vi "TimeTag_Nov 15_2022 - delay adjust.vi"() -> ()   [LabVIEW 2015]
doc: "This sample project is built upon the standard state machine template and shows how you could create an application that acquires, analyzes, and presents data. It includes functionality for presenting configuration dialogs, preserving settings between executions, loading and saving data, as well as exporting graph images and text files.\n\nIt is most appropriate for data that is acquired instantly as it does not allow for screen updates mid acquisition nor does it allow for continuous streaming to disk."
uses:
  <vilib>/ptbypt/NI_PtbyPt.lvlib
panel:
  out "real coin cps 100 pt\n avg 2":dbl
  out "real coin cps 100 pt\n avg SD":dbl
  out "Ch4 100sec avg":dbl
  out "Ch2 100 sec avg":dbl
  out "real coin cps 100 pt\n avg":dbl
  out "all coin cps":dbl
  out "real coin cps":dbl
  out "random coin cps":dbl
  out "Real coin cps":dbl(graph)
  out "total coin/sec - total random coin/sec":dbl
  out "total random coincidences/sec":dbl
  out "Total Coin per sec":dbl
  out "Ch2/4 coin/sec":dbl(graph)
  out "Ch2/4 Total Coincidences":dbl
  out "Channel 2 CPS":dbl(graph)
  out "Channel 4 CPS":dbl(graph)
  out "Total Ch2 CPS":dbl
  out "Total Ch4 CPS":dbl
  in  "Averaging":dbl=10.0
  in  "Runs":dbl=100.0
  in  "Pulse TTL 2":bool
  in  "Pulse TTL 1":bool
  in  "Toggle\nTTL 2":bool
  in  "Toggle\nTTL 1":bool
  out "Total Starts":dbl
  in  "Record data":bool
  out "Initial time":dbl
  out "Elapsed time (s)":dbl
  out "FPGA_Run Status":dbl
  out "USB_Open Status":dbl
  out "Channel 4 Total\nCounts":dbl
  out "Channel 3 Total\nCounts":dbl
  out "Channel 2 Total\nCounts":dbl
  out "Channel 1 Total\nCounts":dbl
  in  "File Name":string="C:\\FPGA\\test.txt"
  out "?":dbl
  out "?":dbl
  out "?":dbl
  out "?":dbl
  out "stats":i64[](array[numeric])
  in  "Stop":bool
  out "Channel 4 CPS":dbl(knob) scale=0.0..2000000.0
  out "Channel 3 CPS":dbl(knob) scale=0.0..600.0
  out "Channel 2 CPS":dbl(knob) scale=0.0..700.0
  out "Channel 1 CPS":dbl(knob) scale=0.0..600.0
  # "Starts"
  # "Channel 1"
  # "Channel 2"
  # "Channel 3"
  # "Channel 4"
  # "Coincidence Channels 1 & 2"
  # "Coincidence Channels 1 & 3"
  # "Coincidence Channels 1 & 4"
  # "Coincidence Channels 2 & 3"
  # "Coincidence Channels 2 & 4"
  # "Coincidence Channels 3 & 4"
  # "Coincidence Channels 1 & 2 & 3"
  # "Coincidence Channels 1 & 2 & 4"
  # "Coincidence Channels 1 & 3 & 4"
  # "Coincidence Channels 2 & 3 & 4"
  # "C:\\FPGA_Lauren"
  # "Coincidence Channels 1 & 2 & 3 & 4"
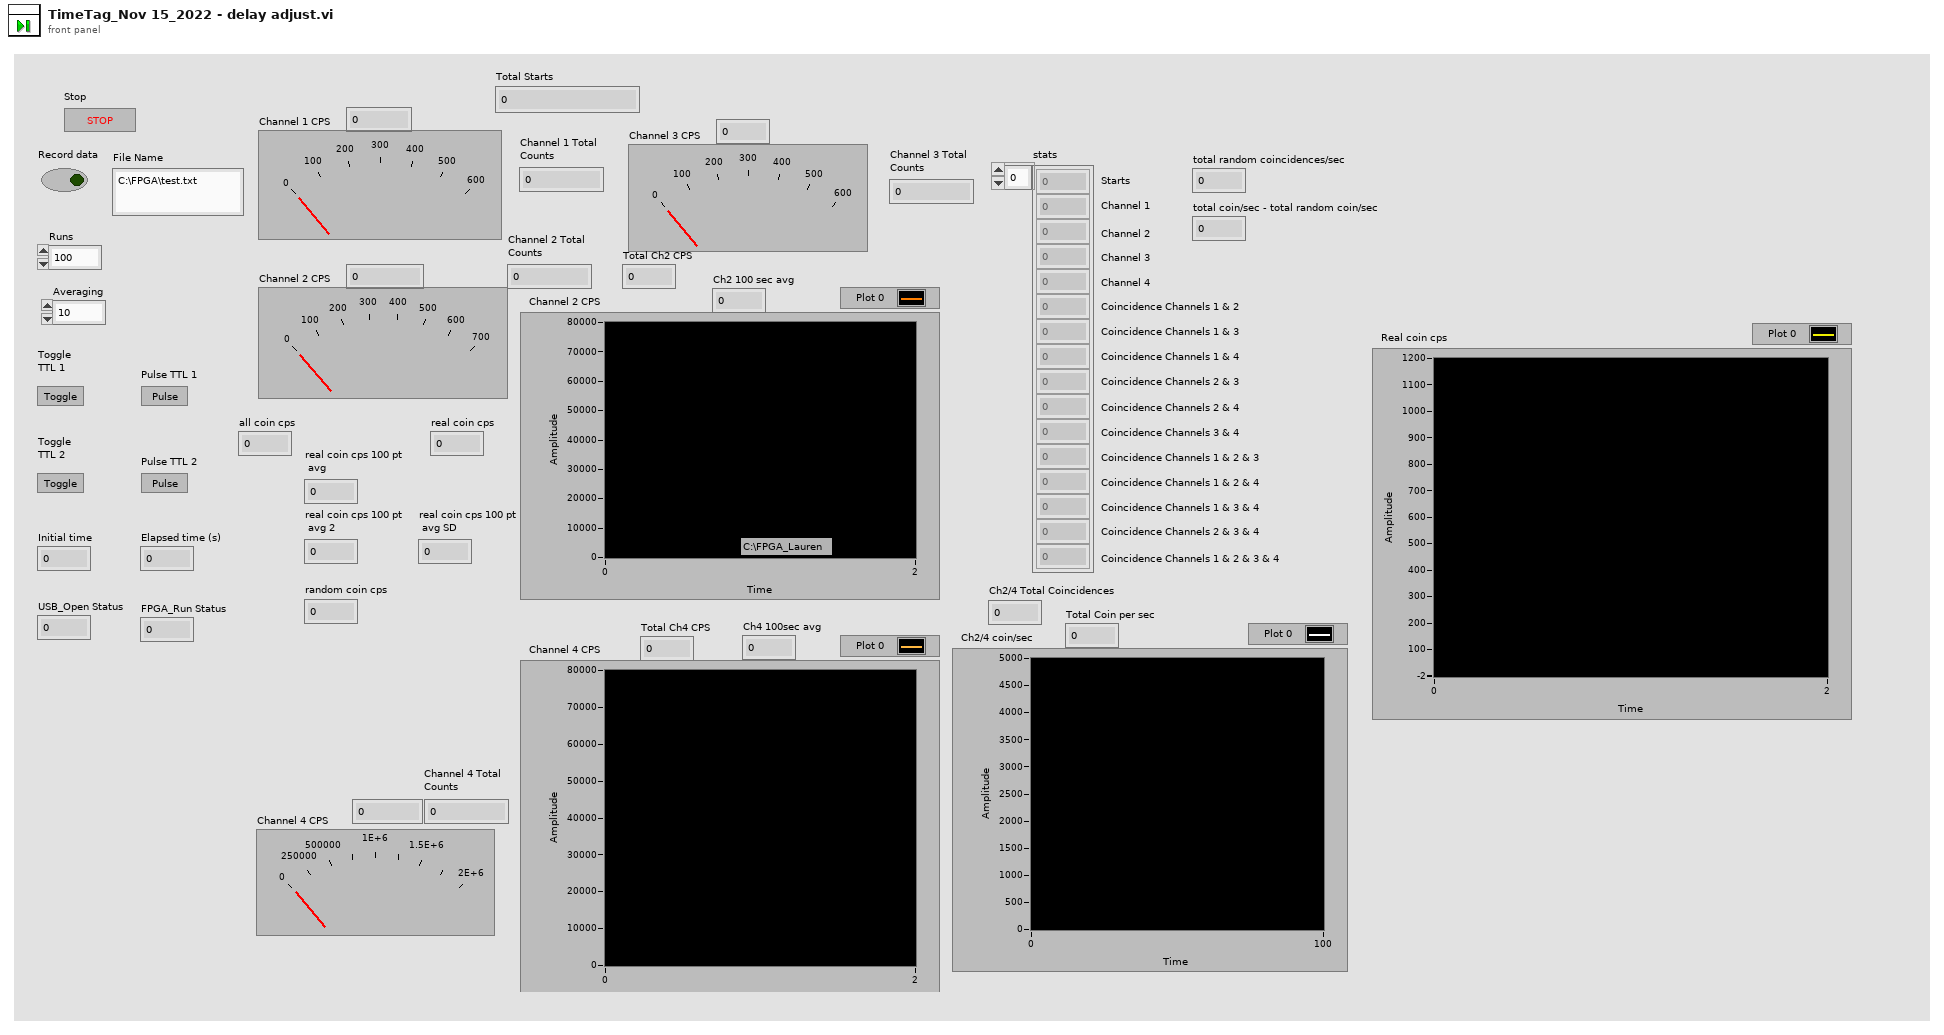
[diagram p1: front panel]
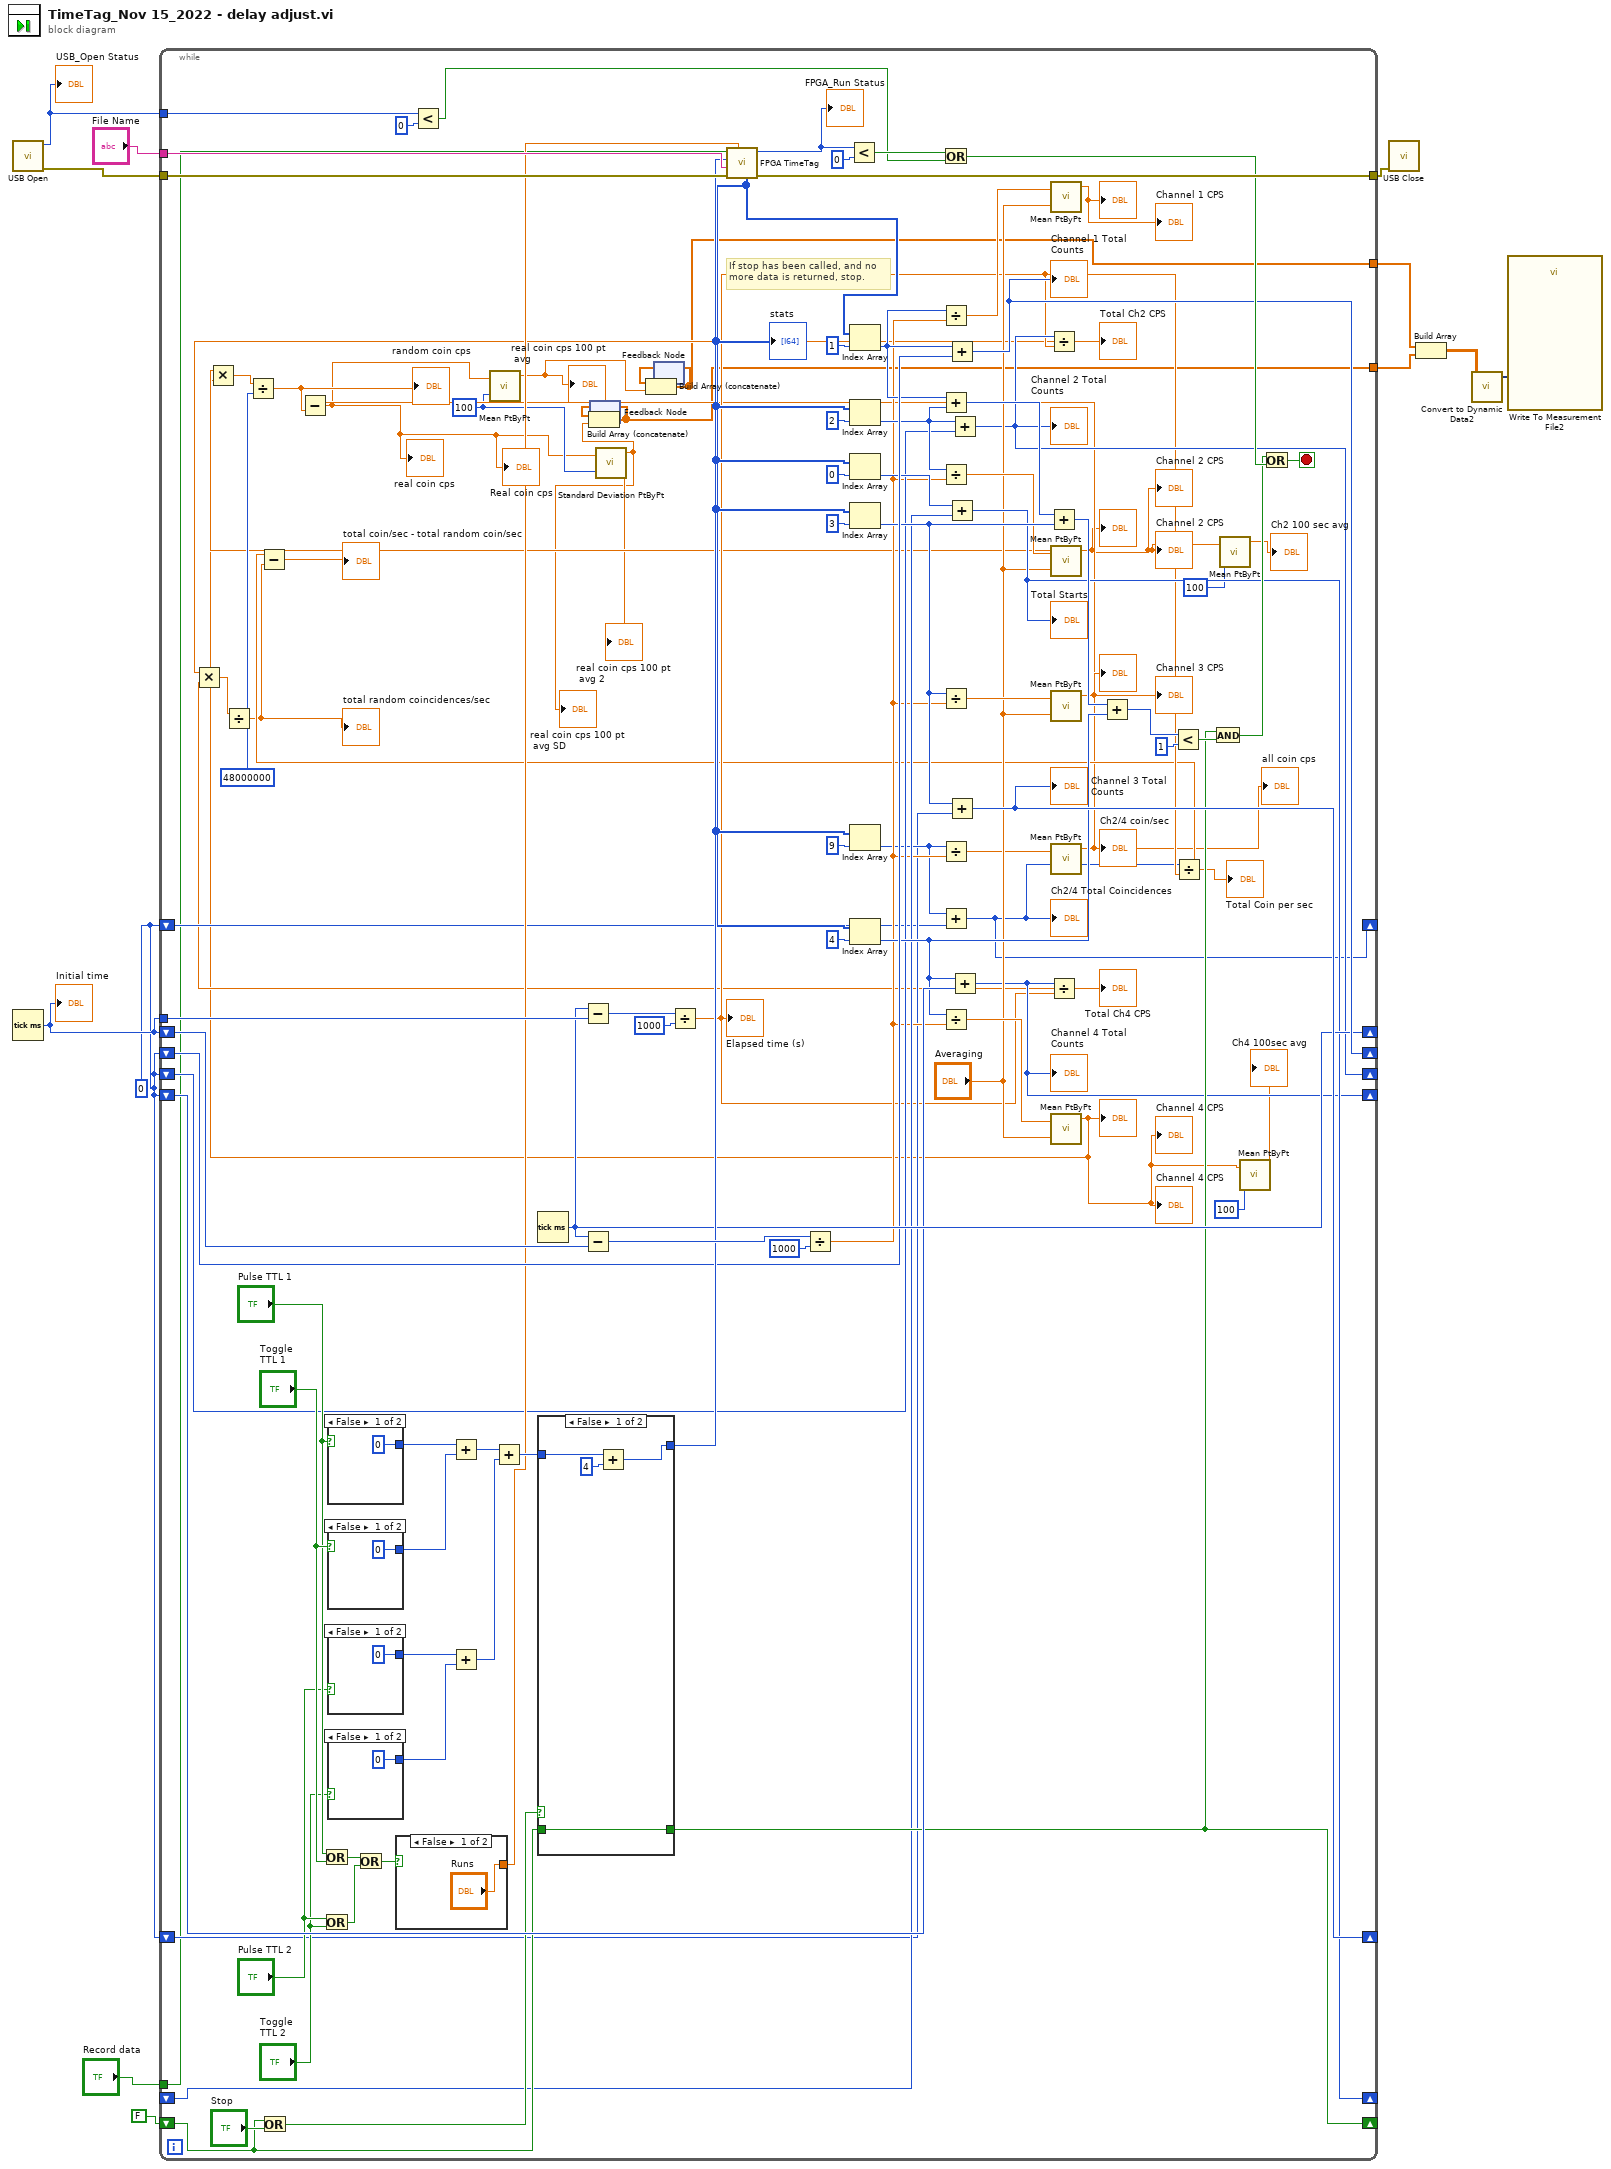
[diagram p0: block diagram]
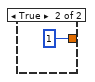
[diagram p2: hidden frame]
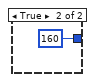
[diagram p3: hidden frame]
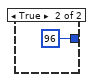
[diagram p4: hidden frame]
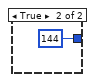
[diagram p5: hidden frame]
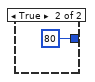
[diagram p6: hidden frame]
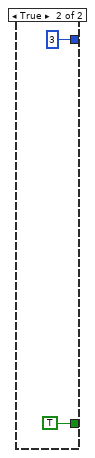
[diagram p7: hidden frame]
diagram:
  w5 = 0
  n1 = call "USB Open.vi"() -> ("error out"=w10:errorcluster, "function return"=w7:i32)  [unwired: 10 in]
  "USB_Open Status" <- w7
  n2 = Tick Count (ms)() -> (millisecond timer value=w8:u32)
  "Initial time" <- w8
  n3 = while {
    tunnel: w8 -> [w117]
    shift-right: [w96] -> _
    shift-left: w5 -> [w92]
    shift-right: [w50] -> _
    shift-left: w5 -> [w46]
    shift-right: [w95] -> _
    shift-left: w5 -> [w42]
    shift-right: [w51] -> _
    shift-left: w5 -> [w91]
    tunnel: w10 -> [w107]
    tunnel: [w108] -> w9
    tunnel: "Record data" -> [w22]
    tunnel: "File Name" -> [w106]
    shift-right: [w93] -> _
    shift-left: w8 -> [w104]
    tunnel: w7 -> [w100]
    shift-right: [w80] -> _
    shift-left: FALSE -> [w77]
    shift-right: [w73] -> _
    shift-left: _ -> [w74]
    shift-right: [w39] -> _
    shift-left: w5 -> [w41]
    tunnel: [w19] -> w4
    tunnel: [w18] -> w3
    stop <- w109 stop-if-true
    w16 = 100
    w33 = 48000000
    # "If stop has been called, and no\nmore data is returned, stop."
    n4 = Or(x=w77, y="Stop") -> (x .or. y?=w79:bool)
    n5 = Or(x="Pulse TTL 1", y="Toggle\nTTL 1") -> (x .or. y?=w64:bool)
    n6 = Or(x="Pulse TTL 2", y="Toggle\nTTL 2") -> (x .or. y?=w65:bool)
    n7 = case shown="False" "Pulse TTL 1" {
      tunnel: [0 80] -> w72
      frame False {
      }
      frame True {
      }
    }
    n8 = case shown="False" "Toggle\nTTL 1" {
      tunnel: [0 96] -> w71
      frame False {
      }
      frame True {
      }
    }
    n9 = case shown="False" "Pulse TTL 2" {
      tunnel: [0 144] -> w68
      frame False {
      }
      frame True {
      }
    }
    n10 = case shown="False" "Toggle\nTTL 2" {
      tunnel: [0 160] -> w69
      frame False {
      }
      frame True {
      }
    }
    n11 = Or(x=w64, y=w65) -> (x .or. y?=w66:bool)
    n12 = case shown="False" w66 {
      tunnel: ["Runs" 1] -> w62
      frame False {
      }
      frame True {
      }
    }
    n13 = Less?(x=w100, y=0) -> (x < y?=w98:bool)
    n14 = Add(x=w72, y=w71) -> (x+y=w70:i32)
    n15 = Add(x=w68, y=w69) -> (x+y=w67:i32)
    n16 = Add(x=w70, y=w67) -> (x+y=w63:i32)
    n17 = Tick Count (ms)() -> (millisecond timer value=w93:u32)
    n18 = case shown="False" w79 {
      tunnel: [w129 3] -> w94
      tunnel: [w131 TRUE] -> w80
      tunnel: w77 -> [w131 _]
      tunnel: w63 -> [w128 _]
      frame False {
        n19 = Add(x=w128, y=4) -> (x+y=w129:i32)
      }
      frame True {
      }
    }
    n20 = Subtract(x=w93, y=w117) -> (x-y=w116:u32)
    n21 = Subtract(x=w93, y=w104) -> (x-y=w103:u32)
    n22 = feedback #1() -> (w20:dbl[])  [unwired: 1 in]
    n23 = feedback #2() -> (w21:dbl[])  [unwired: 1 in]
    n24 = Divide(x=w116, y=1000) -> (x/y=w40:dbl)
    "Elapsed time (s)" <- w40
    n25 = call "FPGA TimeTag.vi"("runs"=w62, "error in (no error)"=w107, "fileName"=w106, "fpgaCommand"=w94, "saveData"=w22) -> ("error out"=w108:errorcluster, "function return"=w105:i32, "stats"=w48:i64[])  [unwired: 4 in]
    "stats" <- w48
    "FPGA_Run Status" <- w105
    n26 = Divide(x=w103, y=1000) -> (x/y=w45:dbl)
    n27 = Less?(x=w105, y=0) -> (x < y?=w99:bool)
    n28 = Index Array(array=w48, index=1) -> (element=w83:i64)
    n29 = Index Array(array=w48, index=2) -> (element=w90:i64)
    n30 = Index Array(array=w48, index=0) -> (element=w75:i64)
    n31 = Index Array(array=w48, index=3) -> (element=w86:i64)
    n32 = Index Array(array=w48, index=9) -> (element=w43:i64)
    n33 = Index Array(array=w48, index=4) -> (element=w87:i64)
    n34 = Or(x=w99, y=w98) -> (x .or. y?=w97:bool)
    n35 = Divide(x=w83, y=w45) -> (x/y=w57:dbl)
    n36 = Add(x=w83, y=w90) -> (x+y=w85:i64)
    n37 = Divide(x=w90, y=w45) -> (x/y=w56:dbl)
    n38 = Divide(x=w86, y=w45) -> (x/y=w55:dbl)
    n39 = Divide(x=w43, y=w45) -> (x/y=w44:dbl)
    n40 = Add(x=w43, y=w41) -> (x+y=w39:i64)
    "Ch2/4 Total Coincidences" <- w39
    n41 = Divide(x=w87, y=w45) -> (x/y=w53:dbl)
    n42 = Add(x=w83, y=w92) -> (x+y=w96:i64)
    "Channel 1 Total\nCounts" <- w96
    n43 = Add(x=w75, y=w74) -> (x+y=w73:i64)
    "Total Starts" <- w73
    n44 = Add(x=w86, y=w42) -> (x+y=w95:i64)
    "Channel 3 Total\nCounts" <- w95
    n45 = Add(x=w90, y=w46) -> (x+y=w50:i64)
    "Channel 2 Total\nCounts" <- w50
    n46 = Add(x=w87, y=w91) -> (x+y=w51:i64)
    "Channel 4 Total\nCounts" <- w51
    n47 = Divide(x=w50, y=w40) -> (x/y=w36:dbl)
    "Total Ch2 CPS" <- w36
    n48 = Add(x=w85, y=w86) -> (x+y=w89:i64)
    n49 = Divide(x=w51, y=w40) -> (x/y=w35:dbl)
    "Total Ch4 CPS" <- w35
    n50 = Multiply(x=w36, y=w35) -> (x*y=w34:dbl)
    n51 = Divide(x=w34, y=w33) -> (x/y=w37:dbl)
    "total random coincidences/sec" <- w37
    n52 = call <vilib>:"Mean PtByPt.vi"("x"=w57, "sample length"="Averaging") -> ("mean"=→"Channel 1 CPS" →"?":dbl)  [unwired: 2 in, 1 out]
    n53 = call <vilib>:"Mean PtByPt.vi"("x"=w56, "sample length"="Averaging") -> ("mean"=w28:dbl)  [unwired: 2 in, 1 out]
    "Channel 2 CPS" <- w28
    "?" <- w28
    "Channel 2 CPS" <- w28
    n54 = call <vilib>:"Mean PtByPt.vi"("x"=w55, "sample length"="Averaging") -> ("mean"=→"Channel 3 CPS" →"?":dbl)  [unwired: 2 in, 1 out]
    n55 = call <vilib>:"Mean PtByPt.vi"("x"=w44) -> ("mean"=w29:dbl)  [unwired: 3 in, 1 out]
    "Ch2/4 coin/sec" <- w29
    "all coin cps" <- w29
    n56 = call <vilib>:"Mean PtByPt.vi"("x"=w53, "sample length"="Averaging") -> ("mean"=w25:dbl)  [unwired: 2 in, 1 out]
    "Channel 4 CPS" <- w25
    "?" <- w25
    "Channel 4 CPS" <- w25
    n57 = Multiply(x=w28, y=w25) -> (x*y=w32:dbl)
    n58 = Divide(x=w32, y=w33) -> (x/y=w31:dbl)
    "random coin cps" <- w31
    n59 = Subtract(x=w29, y=w31) -> (x-y=w15:dbl)
    "Real coin cps" <- w15
    "real coin cps" <- w15
    n60 = call <vilib>:"Mean PtByPt.vi"("x"=w15, "sample length"=w16) -> ("mean"=w17:dbl)  [unwired: 2 in, 1 out]
    "real coin cps 100 pt\n avg" <- w17
    n61 = call <vilib>:"Standard Deviation PtByPt.vi"("x"=w15, "sample length"=w16) -> ("standard deviation"=w13:dbl, "mean"=→"real coin cps 100 pt\n avg 2":dbl)  [unwired: 1 in, 1 out]
    "real coin cps 100 pt\n avg SD" <- w13
    n62 = Build Array (concatenate)(w20, w13) -> (w19:dbl[])
    n63 = feedback-in #1(w19) -> ()
    n64 = Build Array (concatenate)(w21, w17) -> (w18:dbl[])
    n65 = feedback-in #2(w18) -> ()
    n66 = Add(x=w89, y=w87) -> (x+y=w88:i64)
    n67 = Less?(x=w88, y=1) -> (x < y?=w82:bool)
    n68 = Divide(x=w39, y=w40) -> (x/y=w38:dbl)
    "Total Coin per sec" <- w38
    n69 = Subtract(x=w38, y=w37) -> (x-y=→"total coin/sec - total random coin/sec":dbl)
    n70 = And(x=w80, y=w82) -> (x .and. y?=w81:bool)
    n71 = call <vilib>:"Mean PtByPt.vi"("x"=w28, "sample length"=100) -> ("mean"=→"Ch2 100 sec avg":dbl)  [unwired: 2 in, 1 out]
    n72 = call <vilib>:"Mean PtByPt.vi"("x"=w25, "sample length"=100) -> ("mean"=→"Ch4 100sec avg":dbl)  [unwired: 2 in, 1 out]
    n73 = Or(x=w81, y=w97) -> (x .or. y?=w109:bool)
  }
  n74 = call "USB Close.vi"("error in (no error)"=w9) -> ()  [unwired: 9 in, 2 out]
  n75 = Build Array(w3, w4) -> (w2:dbl[][])
  n76 = call "Convert to Dynamic Data2"("2D Array"=w2) -> ("Dynamic Data Type"=w1:dynamicdata)  [unwired: 3 in]
  n77 = call "Write To Measurement File2"("Signals"=w1) -> ()  [unwired: 16 in, 3 out]
